vi "Pump Configure Direction.vi"(8 "error in (no error)":errorcluster, 10 "Message Data":variant, 11 "Data Cluster in":T1 {"Pump Info"."Direction" items=["CW", "CCW"]; "Pump Info"."Speed" format="%03.0f"}) -> (0 "error out":errorcluster, 3 "Data Cluster out":T1 {"Pump Info"."Direction" items=["CW", "CCW"]; "Pump Info"."Speed" format="%03.0f"})   [LabVIEW 2020, in "Pump.lvlib"]
uses:
  Pump.lvlib
  Pump Hardware Configuration.ctl
  support/Message Queue/Message Cluster.ctl
  support/HW Message Cluster.ctl
  support/Message Queue/Message Queue.lvlib
  <instrlib>/WM Pump/WM Pump.lvlib
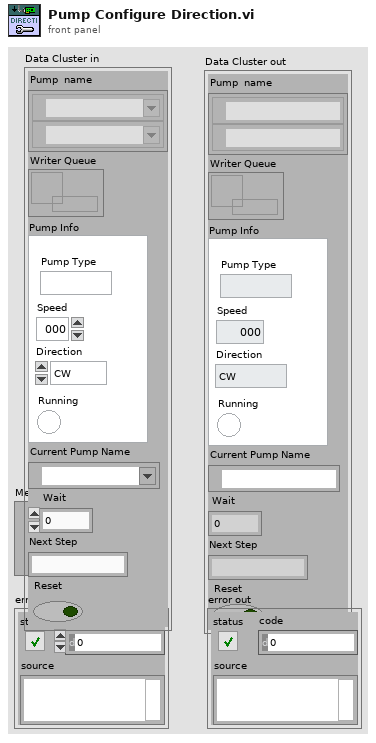
[diagram p1: front panel]
types:
  T1 = typedef "Pump.lvlib/Pump Hardware Configuration.ctl" = cluster{"Pump  name":refnum<visa-resource-name>[], "Writer Queue":refnum<queue>, "Pump Info":cluster{"Pump Type":string, "Speed":i32, "Direction":u16, "Running":bool}, "Current Pump Name":refnum<visa-resource-name>, "Wait":dbl, "Next Step":string, "Reset":bool}
  T2 = typedef "Message Queue.lvlib/HW Message Cluster.ctl" = cluster{"Writer Queue":refnum<queue>, "Writer Data":T3}
  T3 = typedef "Message Queue.lvlib/Message Cluster.ctl" = cluster{"Message":string, "Message Data":variant}
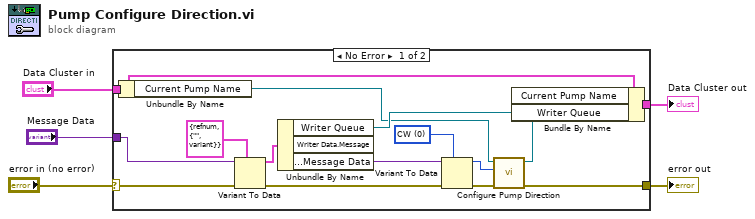
[diagram p0: block diagram]
diagram:
  n1 = case shown="No Error" "error in (no error)" {
    selector: "error in (no error)" -> [w17 w21]
    tunnel: "Message Data" -> [w16 _]
    tunnel: [w20 w22] -> w4
    tunnel: "Data Cluster in" -> [w19 w22]
    tunnel: [w7 w21] -> w2
    frame No Error {
      w11 = u16 0 items=["CW", "CCW"] ("Direction")
      n2 = Unbundle By Name(w19) -> ("Current Pump Name"=w10:refnum<visa-resource-name>)
      n3 = Variant To Data(error in=w17, type=T2 {"Writer Queue"=refnum, "Writer Data"={"Message"="", "Message Data"=variant}}, Variant=w16) -> (data=w18:T2, error out=w13:errorcluster)
      n4 = Unbundle By Name(w18) -> ("Writer Queue"=w15:refnum<queue>, "Writer Data.Message Data"=w12:variant)  [unwired: 1 out]
      n5 = Variant To Data(error in=w13, type=w11, Variant=w12) -> (data=w9:u16, error out=w8:errorcluster)
      n6 = call <instrlib>:"Configure Pump Direction.vi"("error in (no error)"=w8, "Direction"=w9, "VISA resource name"=w10) -> ("error out"=w7:errorcluster, "VISA resource name out"=w6:refnum<visa-resource-name>)  [unwired: 7 in]
      n7 = Bundle By Name(cluster=w19, "Current Pump Name"=w6, "Writer Queue"=w15) -> (w20:T1)
    }
    frame Error {
    }
  }
  "Data Cluster out" <- w4
  "error out" <- w2
